vi "ArraySizeEqualizer.vi"(0 "Array1in":dbl[](array[numeric]), 1 "Array 2in":dbl[](array[numeric])) -> (2 "Array1out":dbl[](array[numeric]), 3 "Array2out":dbl[](array[numeric]), 4 "Numeric":i32)   [LabVIEW 2015]
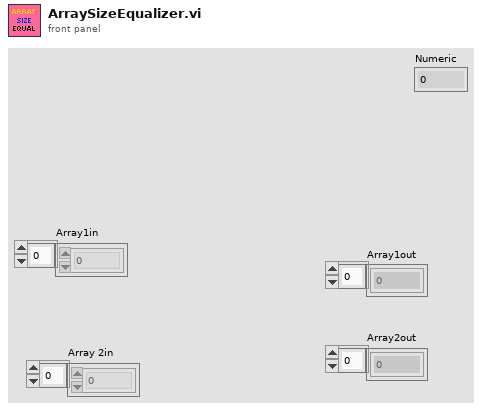
[diagram p1: front panel]
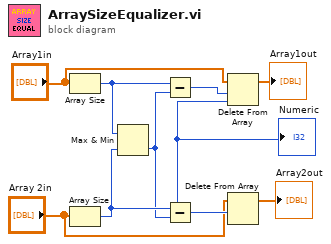
[diagram p0: block diagram]
diagram:
  n1 = Array Size(array="Array1in") -> (size(s)=w8:i32)
  n2 = Array Size(array="Array 2in") -> (size(s)=w3:i32)
  n3 = Max & Min(x=w8, y=w3) -> (min(x,y)=w1:i32)  [unwired: 1 out]
  "Numeric" <- w1
  n4 = Subtract(x=w8, y=w1) -> (x-y=w7:i32)
  n5 = Subtract(x=w3, y=w1) -> (x-y=w5:i32)
  n6 = Delete From Array(array="Array1in", length=w7, index=w1) -> (array with subset deleted=→"Array1out":dbl[])  [unwired: 1 out]
  n7 = Delete From Array(array="Array 2in", length=w5) -> (array with subset deleted=→"Array2out":dbl[])  [unwired: 1 in, 1 out]
